vi "Pad array with wrap around data (U8).vi"(9 "Extra wrap around data (5%)":dbl=5.0 min=5.0 max=100.0, 11 "Array":u8[][](array[numeric])) -> (1 "Pad Size":i32, 2 "Original Size":i32, 3 "Padded Array":u8[][](array[numeric]))   [LabVIEW 2010]
doc: "Wraps 2-D array data by specified percent. REENTRANT to allow parallel non blocking calls."
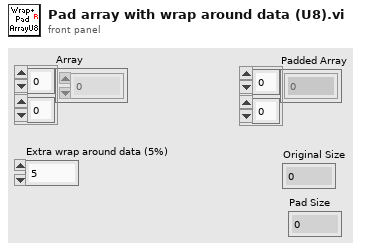
[diagram p1: front panel]
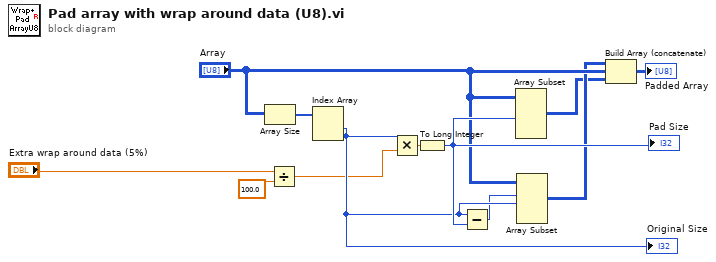
[diagram p0: block diagram]
diagram:
  n1 = Array Size(array="Array") -> (size(s)=w1:i32[])
  n2 = Divide(x="Extra wrap around data (5%)", y=100.0) -> (x/y=w6:dbl)
  n3 = Index Array(array=w1) -> (element #1=w9:i32)  [unwired: 2 in, 1 out]
  "Original Size" <- w9
  n4 = Multiply(x=w9, y=w6) -> (x*y=w11:dbl)
  n5 = To Long Integer(number=w11) -> (32bit integer=w12:i32)
  "Pad Size" <- w12
  n6 = Subtract(x=w9, y=w12) -> (x-y=w2:i32)
  n7 = Array Subset(array="Array", length (row)=w12) -> (w3:u8[][])  [unwired: 3 in]
  n8 = Array Subset(array="Array", index (row)=w2, length (row)=w9) -> (w7:u8[][])  [unwired: 2 in]
  n9 = Build Array (concatenate)(w7, "Array", w3) -> (→"Padded Array":u8[][])
